vi "GFGDisplayRefsGet.vi"(7 "GFG Refnum (use when calling from external project)":refnum<vi>, 8 "error in (no error)":errorcluster) -> (0 "error out":errorcluster, 3 "DisplayRefsOut(generic class)":T1)   [LabVIEW 2012, in "GFG library.lvlib"]
doc: "SciScan 1.2 160622"
uses:
  GFG library.lvlib
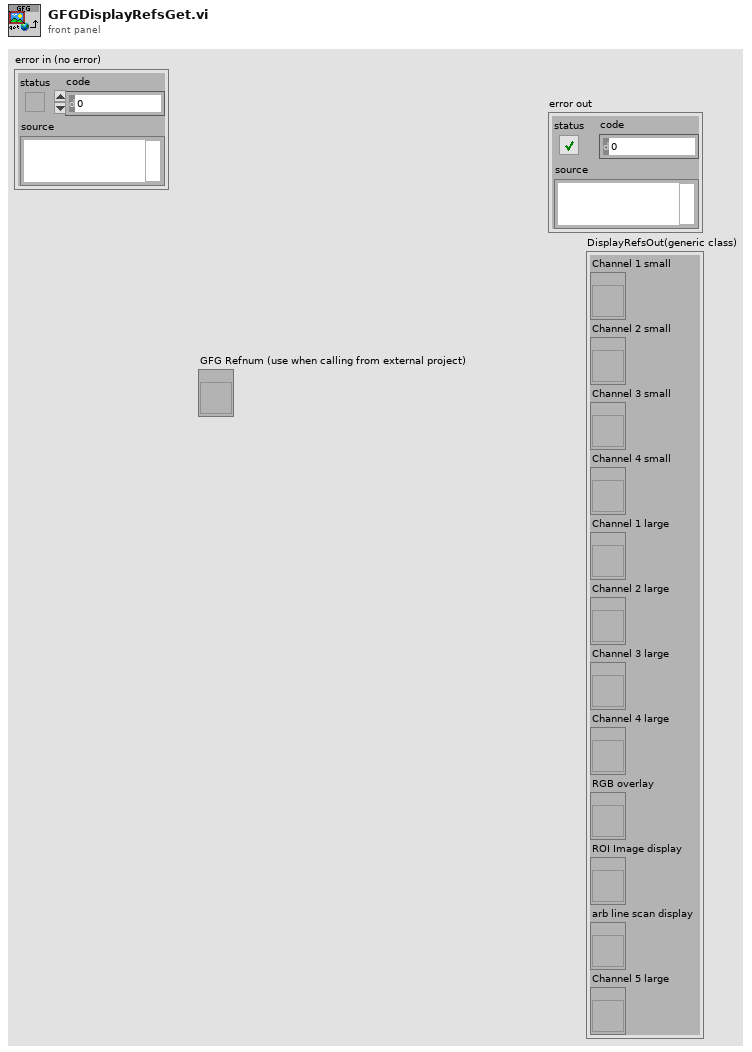
[diagram p1: front panel]
types:
  T1 = cluster{"Channel 1 small":refnum<vi>, "Channel 2 small":refnum<vi>, "Channel 3 small":refnum<vi>, "Channel 4 small":refnum<vi>, "Channel 1 large":refnum<vi>, "Channel 2 large":refnum<vi>, "Channel 3 large":refnum<vi>, "Channel 4 large":refnum<vi>, "RGB overlay":refnum<vi>, "ROI Image display":refnum<vi>, "arb line scan display":refnum<vi>, "Channel 5 large":refnum<vi>}
  T2 = typedef "VariantType.lvlib/Type.ctl" = enum8{"Invalid Type", "Void", "I8", "I16", "I32", "I64", "U8", "U16", "U32", "U64", "Single Float", "Double Float", "Extended Float", "Single Complex", "Double Complex", "Extended Complex", "Enum U8", "Enum U16", "Enum U32", "Enum U64", "Single Float With Unit", "Double Float With Unit", "Extended Float With Unit", "Single Complex with Unit", "Double Complex with Unit", "Extended Complex with Unit", "Boolean", "String", "Path", "Picture", "Tag", "Array", "Cluster", "Variant", "LV Variant", "Waveform", "Timestamp", "Digital Waveform", "Digital Data", "ExpressData", "Refnum", "External Data", "VI", "Poly VI", "LabVIEW Class Instance", "Fixed Point"}
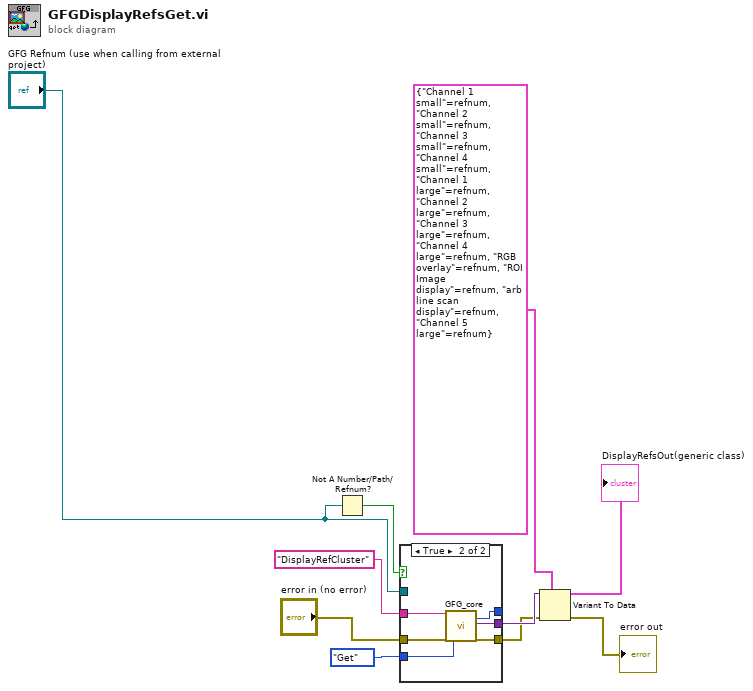
[diagram p0: block diagram]
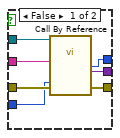
[diagram p2: hidden frame]
diagram:
  n1 = Not A Number/Path/Refnum?(number/path/refnum="GFG Refnum (use when calling from external project)") -> (NaN/Path/Refnum?=w7:bool)
  n2 = case shown="True" w7 {
    tunnel: enum16{"Init", "Set", "Get"}."Get" ("Action") -> [w12 w23]
    tunnel: "DisplayRefCluster" ("Variable Name in") -> [w13 w22]
    tunnel: "error in (no error)" -> [w17 w21]
    tunnel: [w16 w20] -> w3
    tunnel: [w14 w19] -> _
    tunnel: [w15 w18] -> w4
    tunnel: "GFG Refnum (use when calling from external project)" -> [w11 _]
    frame False {
      n3 = call-by-ref "?"(reference=w11, "Variable Name in"=w13, "error in (no error)"=w17, "Action"=w12) -> ("Data Type Out"=w14:T2, "Variant Out"=w15:variant, "error out"=w16:errorcluster)  [unwired: 11 in, 6 out]
    }
    frame True {
      n4 = call "GFG_core.vi"("Variable Name in"=w22, "error in (no error)"=w21, "Action"=w23) -> ("Data Type Out"=w19:T2, "Variant Out"=w18:variant, "error out"=w20:errorcluster)  [unwired: 10 in, 4 out]
    }
  }
  n5 = Variant To Data(error in=w3, type=T1 {"Channel 1 small"=refnum, "Channel 2 small"=refnum, "Channel 3 small"=refnum, "Channel 4 small"=refnum, "Channel 1 large"=refnum, "Channel 2 large"=refnum, "Channel 3 large"=refnum, "Channel 4 large"=refnum, "RGB overlay"=refnum, "ROI Image display"=refnum, "arb line scan display"=refnum, "Channel 5 large"=refnum} ("display refs cluster"), Variant=w4) -> (data=→"DisplayRefsOut(generic class)":T1, error out=→"error out":errorcluster)
